vi "ZedBoardWordCalculator.vi"() -> ()   [LabVIEW 2012]
panel:
  in  "Power Pulse\nReject Config":u16
  in  "Power Mon \nAcc Mode":string(combo)
  in  "Power Mon Test Mode":string(combo)
  in  "0       1   ...    Power Mon Chan Enable    ...      9       10     11":bool[](array[boolean])
  out "word9":string
  in  "SoftDEMUX \nSelector Enable":bool
  in  "Sync Select 3B":string(combo)
  in  "Sync Select 2B":string(combo)
  in  "Sync Select 1B":string(combo)
  in  "Sync Select 0B":string(combo)
  in  "Sync Select 7":string(combo)
  in  "Sync Select 6":string(combo)
  in  "Sync Select 5":string(combo)
  in  "Sync Select 4":string(combo)
  in  "Sync Select 3A":string(combo)
  in  "Sync Select 2A":string(combo)
  in  "Sync Select 1A":string(combo)
  in  "Sync Select 0A":string(combo)
  in  "Sync Test\nMode Config":u32
  in  "Pulse Period\n(clock cycles -1)":u32
  in  "Channel DEMUX \nSelector":bool
  in  "Channel \nHold Order":bool
  in  "Channel \nTransfer Order":bool
  in  "Throttle Mode":string(combo)
  in  "Sync Test Mode Select":string(combo)
  in  "Data Input Test Mode":string(combo)
  in  "PIN5 Pulse Durration Ave 2^N":u16
  in  "PIN4 Pulse Durration Ave 2^N":u16
  in  "PIN3 Pulse Durration Ave 2^N":u16
  in  "PIN2 Pulse Durration Ave 2^N":u16
  in  "PIN1 Pulse Durration Ave 2^N":u16
  out "wordA":string
  in  "PIN0 Pulse Durration Ave 2^N":u16
  in  "Sync Input Polarity":bool[](array[boolean])
  in  "DIN Demux Polarity":bool[](array[boolean])
  in  "DIN Polarity":bool[](array[boolean])
  out "word8":string
  out "word7":string
  out "word6":string
  out "word5":string
  out "word4":string
  out "word3":string
  out "word2":string
  out "word1":string
  out "word0":string
  in  "Demux Channel Enable":bool[](array[boolean])
  in  "Relative Time Step":u32
  in  "Time Reset":bool
  in  "Profiles Per Histogram":u16
  in  "Number of Bins":u16
  in  "User Reset":bool
  in  "Counts Per Bin":u16
  in  "0      1       2   ...    Reset Profile Accumulator     ...   10     11":bool[](array[boolean])
  in  "0       1      2    ...     Channel Enable        ...         9      10     11":bool[](array[boolean])
  in  "Sync Enable":bool[](array[boolean])
  in  "stop":bool
  # "word0"
  # "word1"
  # "word2"
  # "word3"
  # "word4"
  # "valid range (2-4096)"
  # "valid range (2-4096)"
  # "valid range (1-32,768)"
  # "word5"
  # "word6"
  # "valid range (0-64)"
  # "valid range (0-256)"
  # "word7"
  # "word8"
  # "word9"
  # "valid range (0-256)"
  # "wordA"
  # "N=valid range (0-15)"
  # "N=valid range (0-15)"
  # "N=valid range (0-15)"
  # "N=valid range (0-15)"
  # "N=valid range (0-15)"
  # "N=valid range (0-15)"
  # "word0"
  # "word1"
  # "word2"
  # "word3"
  # "word4"
  # "valid range (2-4096)"
  # "valid range (2-4096)"
  # "valid range (1-32,768)"
  # "word5"
  # "word6"
  # "valid range (0-256)"
  # "valid range (0-64)"
  # "word7"
  # "word8"
  # "valid range (0-33,554,432)"
  # "word9"
  # "N=valid range (0-15)"
  # "N=valid range (0-15)"
  # "N=valid range (0-15)"
  # "N=valid range (0-15)"
  # "N=valid range (0-15)"
  # "N=valid range (0-15)"
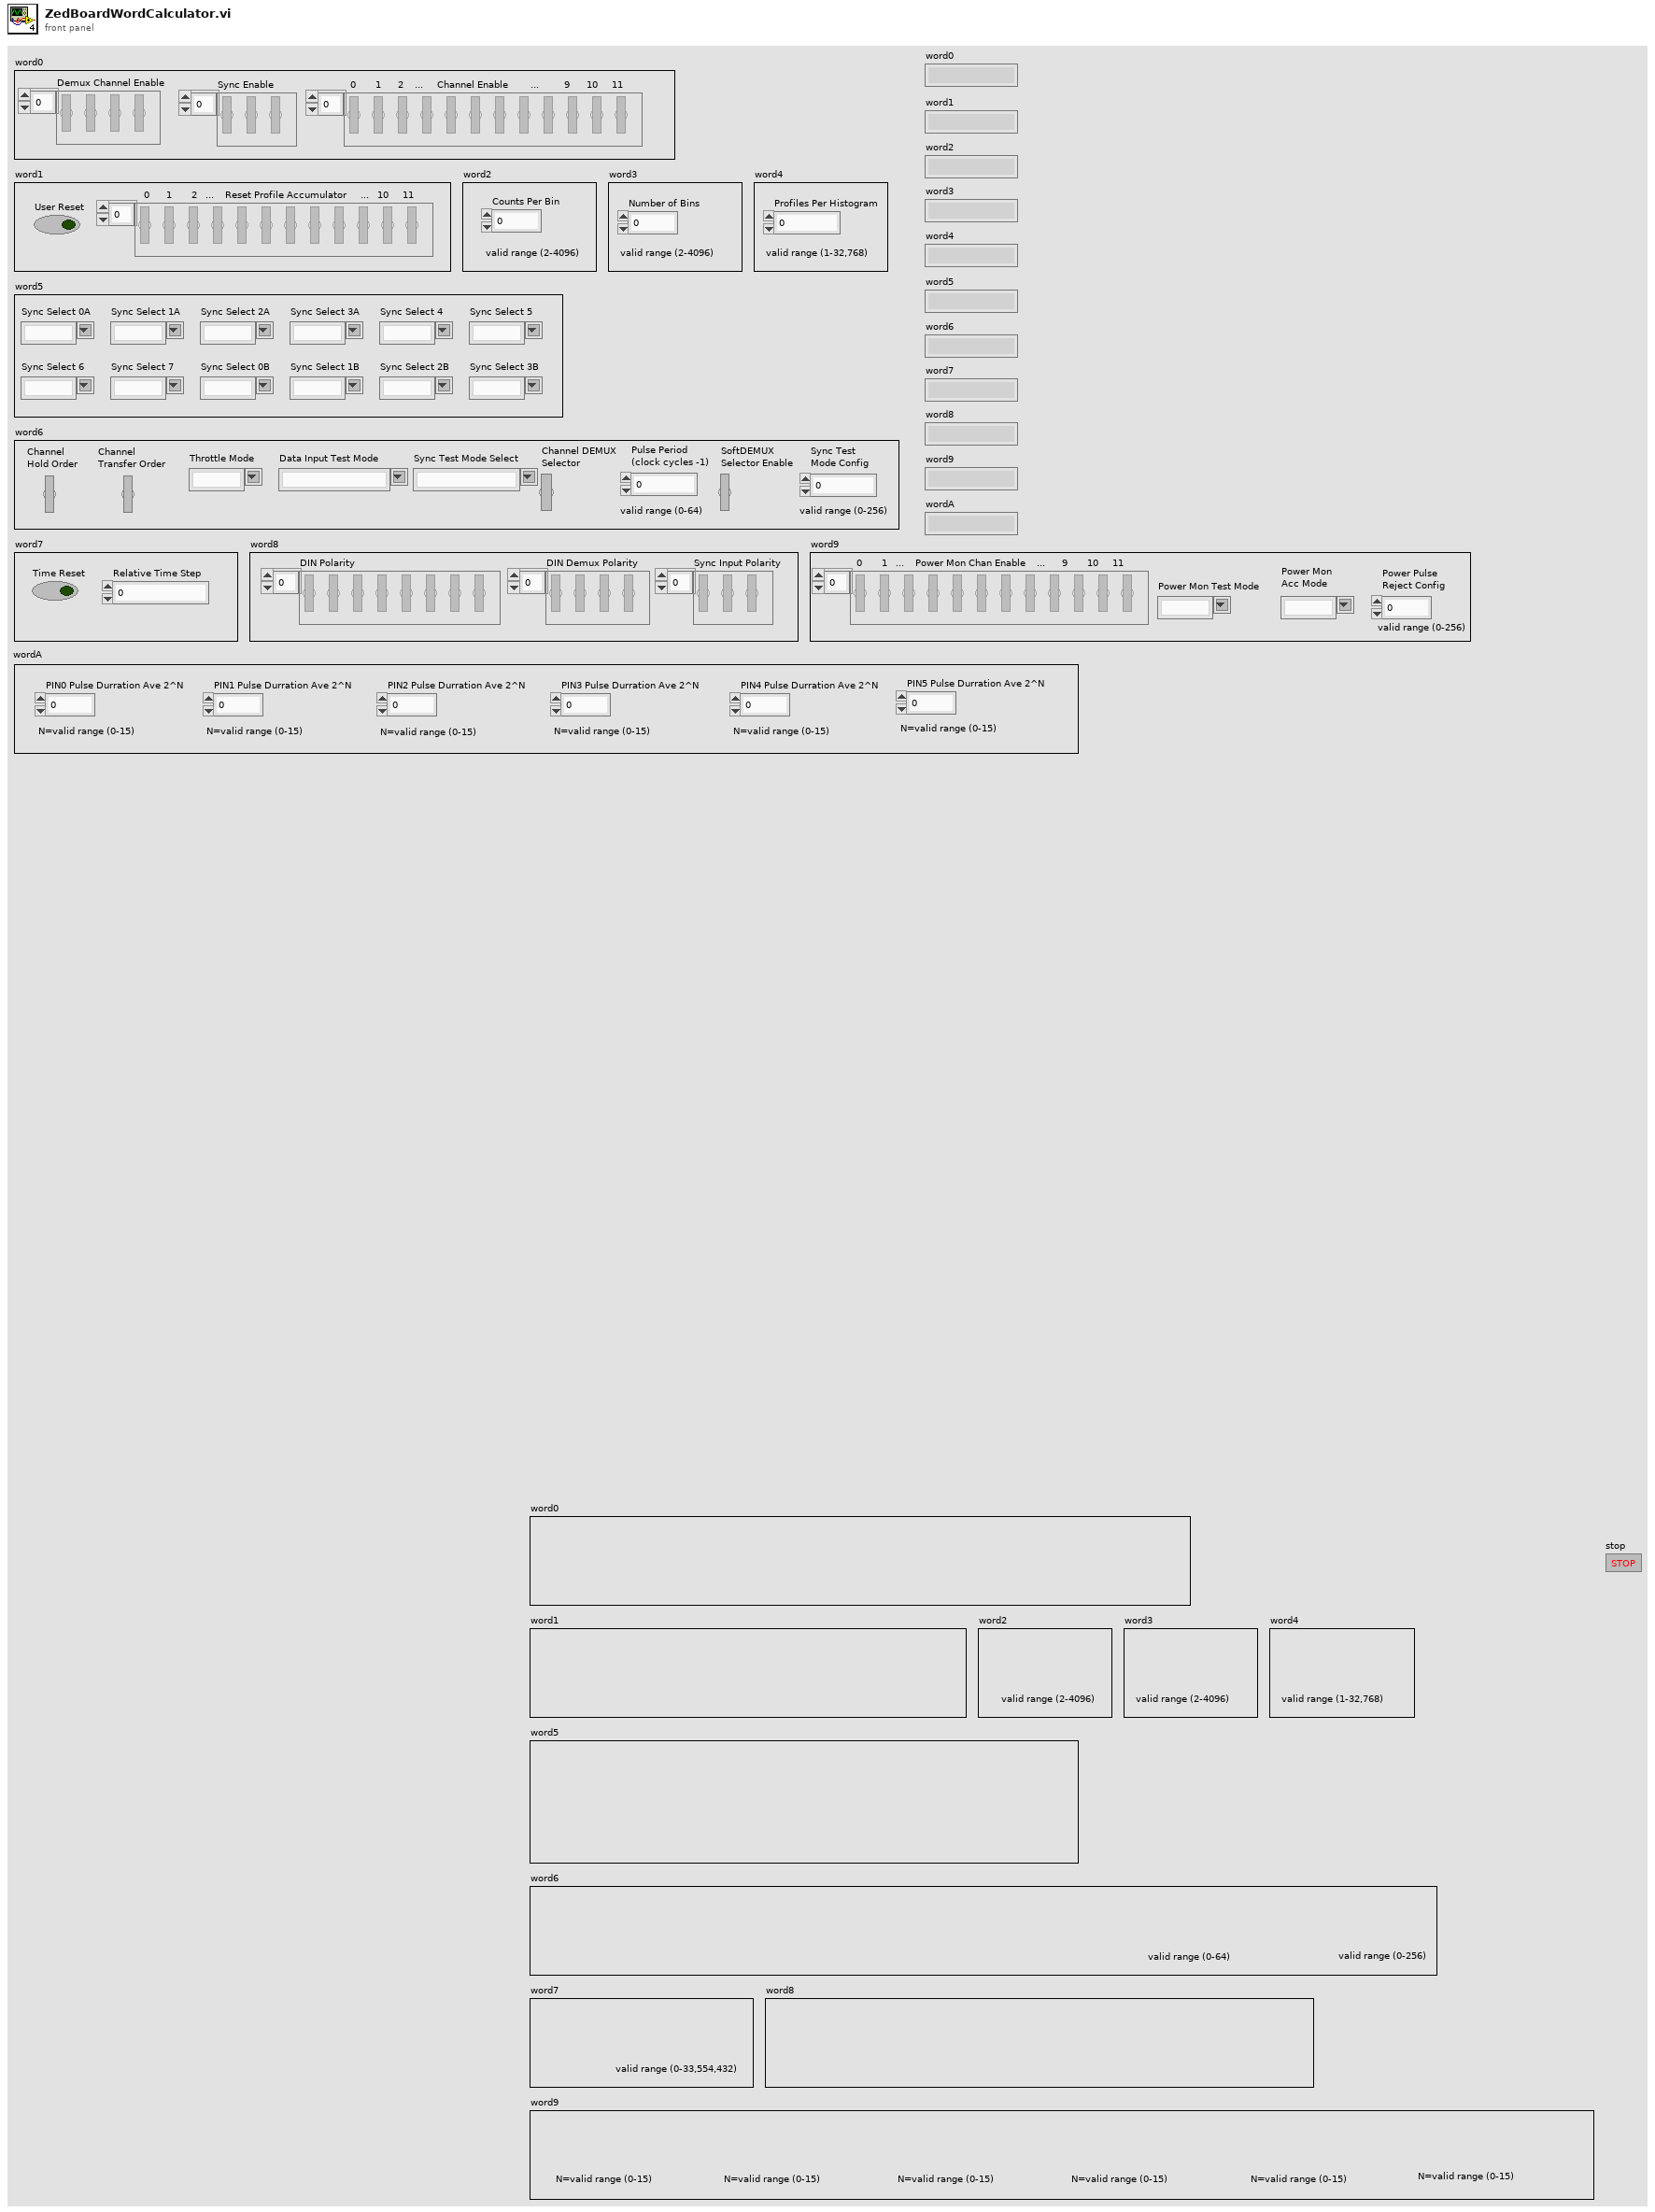
[diagram p1: front panel]
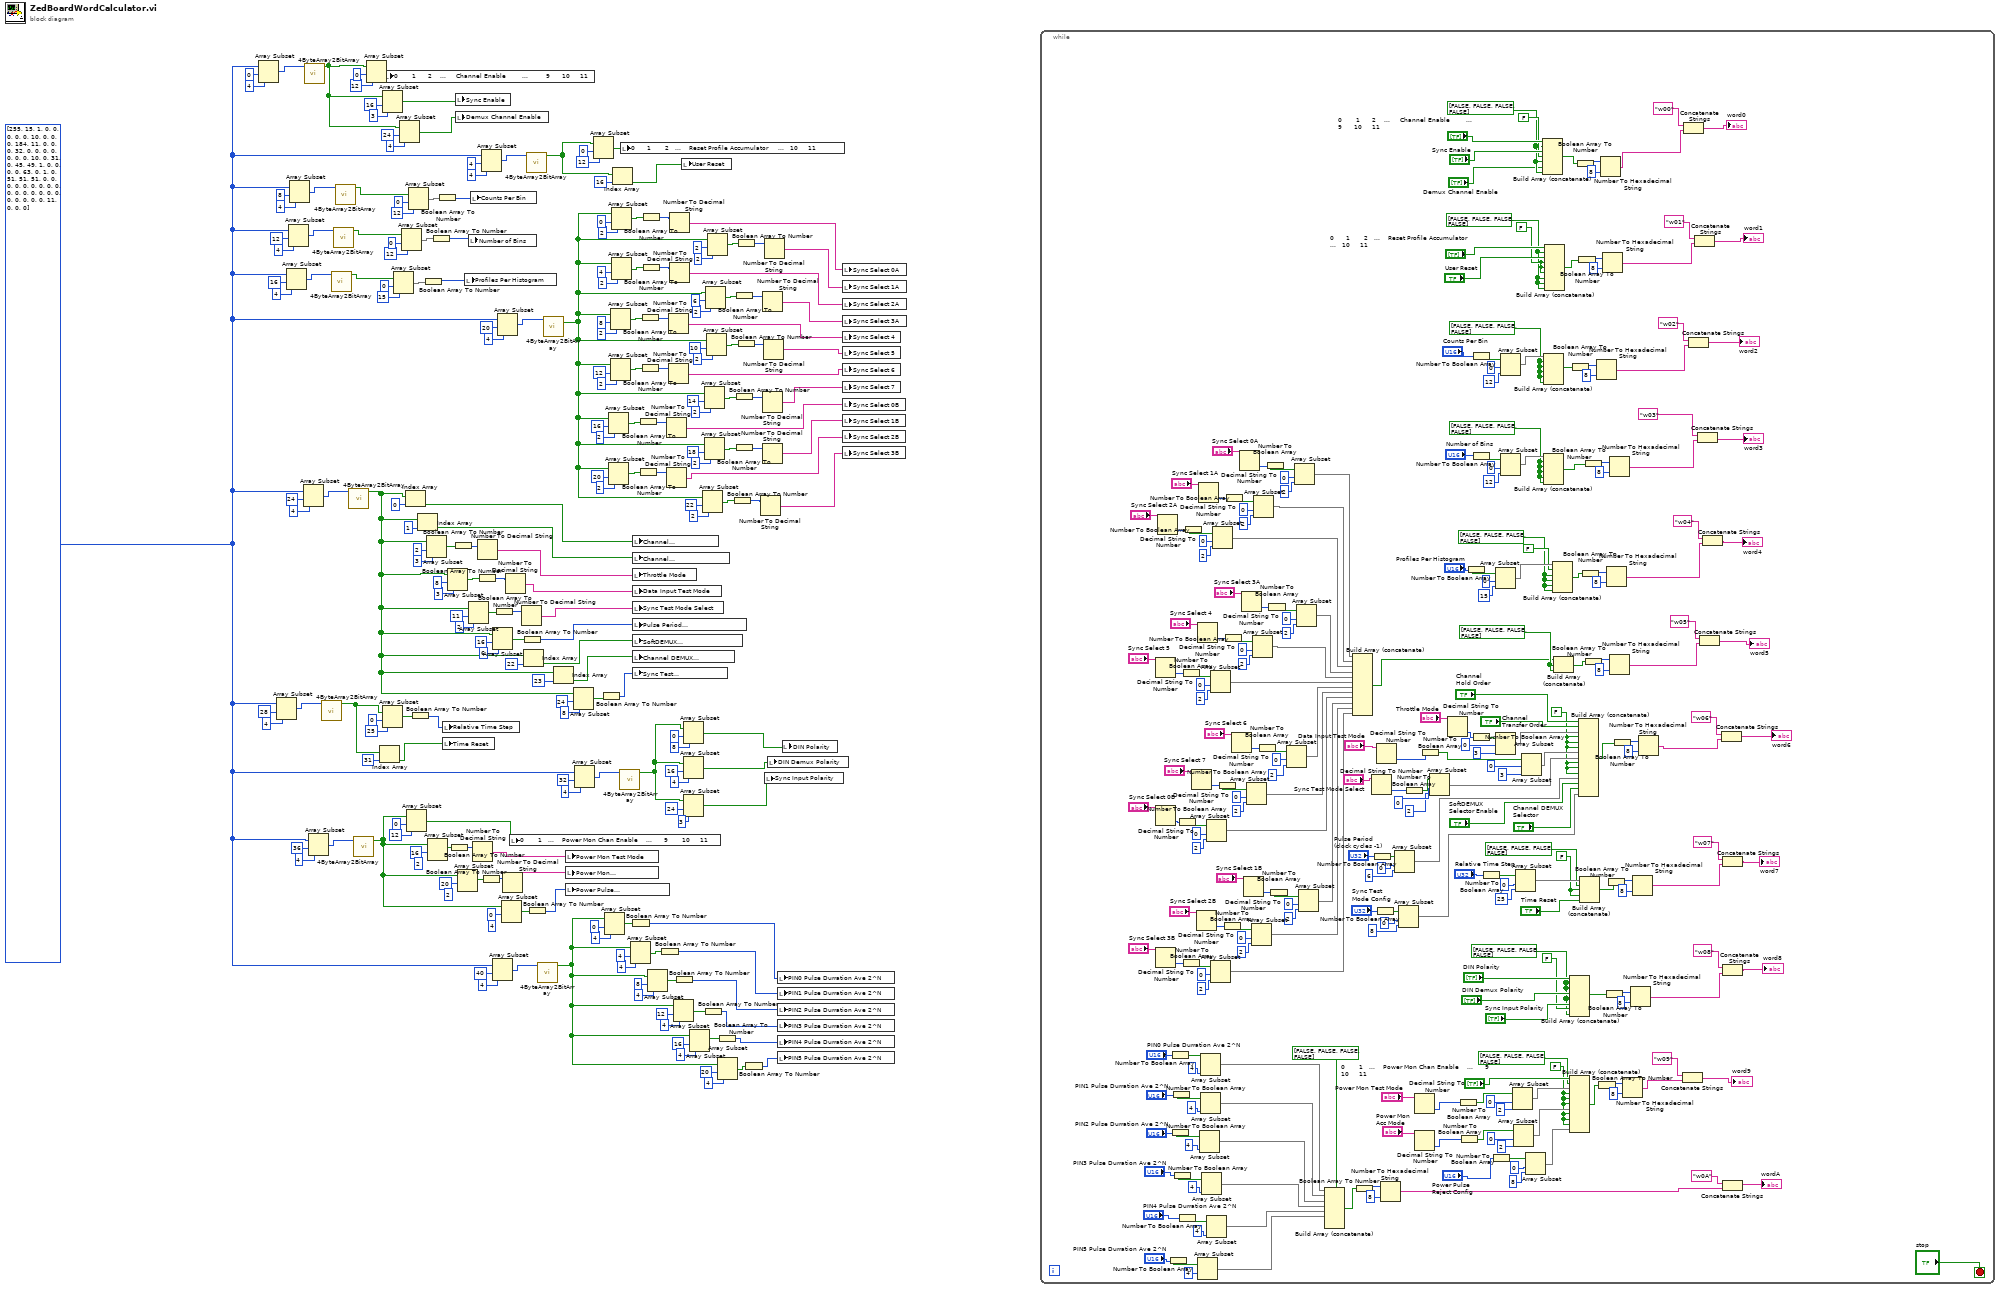
[diagram p0: block diagram]
diagram:
  (unwired) 4 ("length")
  (unwired) 2 ("length")
  (unwired) 2 ("length")
  w1 = u8[] [255, 15, 1, 0, 0, 0, 0, 0, 10, 0, 0, 0, 184, 11, 0, 0, 0, 32, 0, 0, 0, 0, 0, 0, 0, 10, 0, 31, 0, 45, 49, 1, 0, 0, 0, 0, 63, 0, 1, 0, 51, 51, 51, 0, 0, 0, 0, 0, 0, 0, 0, 0, 0, 0, 0, 0, 0, 0, 0, 0, 0, 0, 0, 0, 11, 0, 0, 0] ("subarray")
  n1 = Array Subset(array=w1, index=0, length=4) -> (w183:u8[])
  n2 = Array Subset(array=w1, index=28, length=4) -> (w189:u8[])
  n3 = Array Subset(array=w1, index=16, length=4) -> (w198:u8[])
  n4 = Array Subset(array=w1, index=12, length=4) -> (w201:u8[])
  n5 = Array Subset(array=w1, index=8, length=4) -> (w204:u8[])
  n6 = Array Subset(array=w1, index=24, length=4) -> (w192:u8[])
  n7 = call "4ByteArray2BitArray.vi"("array"=w183) -> ("Array"=w25:bool[])  [unwired: 10 in]
  n8 = Array Subset(array=w1, index=36, length=4) -> (w17:u8[])
  n9 = call "4ByteArray2BitArray.vi"("array"=w189) -> ("Array"=w145:bool[])  [unwired: 10 in]
  n10 = call "4ByteArray2BitArray.vi"("array"=w198) -> ("Array"=w47:bool[])  [unwired: 10 in]
  n11 = call "4ByteArray2BitArray.vi"("array"=w201) -> ("Array"=w42:bool[])  [unwired: 10 in]
  n12 = call "4ByteArray2BitArray.vi"("array"=w204) -> ("Array"=w37:bool[])  [unwired: 10 in]
  n13 = call "4ByteArray2BitArray.vi"("array"=w192) -> ("Array"=w22:bool[])  [unwired: 10 in]
  n14 = call "4ByteArray2BitArray.vi"("array"=w17) -> ("Array"=w3:bool[])  [unwired: 10 in]
  n15 = Array Subset(array=w25, index=0, length=12) -> (w213:bool[])
  n16 = Index Array(array=w145, index=31) -> (element=w143:bool)
  n17 = Array Subset(array=w25, index=16, length=3) -> (w24:bool[])
  n18 = Array Subset(array=w145, index=0, length=25) -> (w141:bool[])
  n19 = local write "0       1      2    ...     Channel Enable        ...         9      10     11"(w213) -> ()
  n20 = Array Subset(array=w47, index=0, length=15) -> (w48:bool[])
  n21 = Array Subset(array=w25, index=24, length=4) -> (w23:bool[])
  n22 = Array Subset(array=w42, index=0, length=12) -> (w43:bool[])
  n23 = Index Array(array=w22, index=0) -> (element=w123:bool)
  n24 = Array Subset(array=w3, index=0, length=12) -> (w14:bool[])
  n25 = Array Subset(array=w37, index=0, length=12) -> (w38:bool[])
  n26 = Boolean Array To Number(Boolean array=w141) -> (number=w142:u32)
  n27 = Index Array(array=w22, index=1) -> (element=w122:bool)
  n28 = Boolean Array To Number(Boolean array=w48) -> (number=w46:u32)
  n29 = Array Subset(array=w22, index=2, length=3) -> (w129:bool[])
  n30 = Array Subset(array=w3, index=16) -> (w12:bool[])  [unwired: 1 in]
  n31 = Boolean Array To Number(Boolean array=w43) -> (number=w41:u32)
  n32 = Boolean Array To Number(Boolean array=w38) -> (number=w36:u32)
  n33 = local write "Relative Time Step"(w142) -> ()
  n34 = local write "Time Reset"(w143) -> ()
  n35 = Array Subset(array=w22, index=8, length=3) -> (w130:bool[])
  n36 = Boolean Array To Number(Boolean array=w12) -> (number=w11:u32)
  n37 = Boolean Array To Number(Boolean array=w129) -> (number=w121:u32)
  n38 = local write "Sync Enable"(w24) -> ()
  n39 = local write "Demux Channel Enable"(w23) -> ()
  n40 = Array Subset(array=w3, index=20) -> (w8:bool[])  [unwired: 1 in]
  n41 = local write "Profiles Per Histogram"(w46) -> ()
  n42 = local write "Number of Bins"(w41) -> ()
  n43 = Array Subset(array=w22, index=11, length=2) -> (w128:bool[])
  n44 = local write "Counts Per Bin"(w36) -> ()
  n45 = Number To Decimal String(number=w11) -> (decimal integer string=w10:string)  [unwired: 1 in]
  n46 = Boolean Array To Number(Boolean array=w130) -> (number=w119:u32)
  n47 = Number To Decimal String(number=w121) -> (decimal integer string=w120:string)  [unwired: 1 in]
  n48 = Array Subset(array=w1, index=4, length=4) -> (w207:u8[])
  n49 = Boolean Array To Number(Boolean array=w8) -> (number=w7:u32)
  n50 = Array Subset(array=w1, index=40, length=4) -> (w210:u8[])
  n51 = Array Subset(array=w22, index=16, length=6) -> (w127:bool[])
  n52 = Boolean Array To Number(Boolean array=w128) -> (number=w117:u32)
  n53 = Array Subset(array=w1, index=20, length=4) -> (w195:u8[])
  n54 = Array Subset(array=w3, index=0) -> (w4:bool[])  [unwired: 1 in]
  n55 = Number To Decimal String(number=w7) -> (decimal integer string=w6:string)  [unwired: 1 in]
  n56 = Number To Decimal String(number=w119) -> (decimal integer string=w118:string)  [unwired: 1 in]
  n57 = local write "0       1   ...    Power Mon Chan Enable    ...      9       10     11"(w14) -> ()
  n58 = Number To Decimal String(number=w117) -> (decimal integer string=w116:string)  [unwired: 1 in]
  n59 = Boolean Array To Number(Boolean array=w127) -> (number=w113:u32)
  n60 = Index Array(array=w22, index=22) -> (element=w20:bool)
  n61 = call "4ByteArray2BitArray.vi"("array"=w207) -> ("Array"=w32:bool[])  [unwired: 10 in]
  n62 = Boolean Array To Number(Boolean array=w4) -> (number=w2:u32)
  n63 = call "4ByteArray2BitArray.vi"("array"=w210) -> ("Array"=w170:bool[])  [unwired: 10 in]
  n64 = call "4ByteArray2BitArray.vi"("array"=w195) -> ("Array"=w63:bool[])  [unwired: 10 in]
  n65 = Index Array(array=w22, index=23) -> (element=w114:bool)
  n66 = local write "Power Mon \nAcc Mode"(w6) -> ()
  n67 = local write "Power Mon Test Mode"(w10) -> ()
  n68 = local write "Power Pulse\nReject Config"(w2) -> ()
  n69 = Array Subset(array=w22, index=24, length=8) -> (w126:bool[])
  n70 = Array Subset(array=w1, index=32, length=4) -> (w186:u8[])
  n71 = Array Subset(array=w32, index=0, length=12) -> (w31:bool[])
  n72 = Boolean Array To Number(Boolean array=w126) -> (number=w112:u32)
  n73 = Array Subset(array=w170, index=0, length=4) -> (w167:bool[])
  n74 = Array Subset(array=w63, index=16, length=2) -> (w77:bool[])
  n75 = Array Subset(array=w63, index=20, length=2) -> (w69:bool[])
  n76 = Array Subset(array=w63, index=8, length=2) -> (w93:bool[])
  n77 = Array Subset(array=w63, index=12, length=2) -> (w85:bool[])
  n78 = Array Subset(array=w63, index=0, length=2) -> (w109:bool[])
  n79 = Array Subset(array=w63, index=4, length=2) -> (w101:bool[])
  n80 = Index Array(array=w32, index=16) -> (element=w30:bool)
  n81 = call "4ByteArray2BitArray.vi"("array"=w186) -> ("Array"=w151:bool[])  [unwired: 10 in]
  n82 = local write "0      1       2   ...    Reset Profile Accumulator     ...   10     11"(w31) -> ()
  n83 = Array Subset(array=w170, index=4, length=4) -> (w169:bool[])
  n84 = Boolean Array To Number(Boolean array=w167) -> (number=w166:u32)
  n85 = local write "Channel \nHold Order"(w123) -> ()
  n86 = local write "Channel \nTransfer Order"(w122) -> ()
  n87 = local write "Throttle Mode"(w120) -> ()
  n88 = local write "Data Input Test Mode"(w118) -> ()
  n89 = local write "Sync Test Mode Select"(w116) -> ()
  n90 = local write "Pulse Period\n(clock cycles -1)"(w113) -> ()
  n91 = local write "SoftDEMUX \nSelector Enable"(w20) -> ()
  n92 = local write "Channel DEMUX \nSelector"(w114) -> ()
  n93 = local write "Sync Test\nMode Config"(w112) -> ()
  n94 = Boolean Array To Number(Boolean array=w77) -> (number=w76:u32)
  n95 = Boolean Array To Number(Boolean array=w69) -> (number=w68:u32)
  n96 = Boolean Array To Number(Boolean array=w93) -> (number=w92:u32)
  n97 = Boolean Array To Number(Boolean array=w85) -> (number=w84:u32)
  n98 = Boolean Array To Number(Boolean array=w109) -> (number=w108:u32)
  n99 = Boolean Array To Number(Boolean array=w101) -> (number=w100:u32)
  n100 = Array Subset(array=w170, index=8, length=4) -> (w164:bool[])
  n101 = Boolean Array To Number(Boolean array=w169) -> (number=w168:u32)
  n102 = Number To Decimal String(number=w76) -> (decimal integer string=w54:string)  [unwired: 1 in]
  n103 = Number To Decimal String(number=w68) -> (decimal integer string=w52:string)  [unwired: 1 in]
  n104 = Number To Decimal String(number=w92) -> (decimal integer string=w58:string)  [unwired: 1 in]
  n105 = Number To Decimal String(number=w84) -> (decimal integer string=w56:string)  [unwired: 1 in]
  n106 = Number To Decimal String(number=w108) -> (decimal integer string=w62:string)  [unwired: 1 in]
  n107 = Number To Decimal String(number=w100) -> (decimal integer string=w60:string)  [unwired: 1 in]
  n108 = Array Subset(array=w170, index=12, length=4) -> (w163:bool[])
  n109 = Boolean Array To Number(Boolean array=w164) -> (number=w165:u32)
  n110 = local write "User Reset"(w30) -> ()
  n111 = Array Subset(array=w151, index=16, length=4) -> (w148:bool[])
  n112 = Array Subset(array=w151, index=24, length=3) -> (w149:bool[])
  n113 = Array Subset(array=w151, index=0, length=8) -> (w150:bool[])
  n114 = Array Subset(array=w170, index=16, length=4) -> (w162:bool[])
  n115 = Array Subset(array=w63, index=22, length=2) -> (w65:bool[])
  n116 = Boolean Array To Number(Boolean array=w163) -> (number=w158:u32)
  n117 = Array Subset(array=w63, index=14, length=2) -> (w81:bool[])
  n118 = Array Subset(array=w63, index=18, length=2) -> (w73:bool[])
  n119 = Array Subset(array=w63, index=6, length=2) -> (w97:bool[])
  n120 = Array Subset(array=w63, index=10, length=2) -> (w89:bool[])
  n121 = Array Subset(array=w63, index=2, length=2) -> (w105:bool[])
  n122 = Boolean Array To Number(Boolean array=w162) -> (number=w159:u32)
  n123 = Array Subset(array=w170, index=20, length=4) -> (w161:bool[])
  n124 = Boolean Array To Number(Boolean array=w65) -> (number=w64:u32)
  n125 = Boolean Array To Number(Boolean array=w81) -> (number=w80:u32)
  n126 = Boolean Array To Number(Boolean array=w73) -> (number=w72:u32)
  n127 = Boolean Array To Number(Boolean array=w97) -> (number=w96:u32)
  n128 = Boolean Array To Number(Boolean array=w89) -> (number=w88:u32)
  n129 = Boolean Array To Number(Boolean array=w105) -> (number=w104:u32)
  n130 = Boolean Array To Number(Boolean array=w161) -> (number=w160:u32)
  n131 = Number To Decimal String(number=w64) -> (decimal integer string=w51:string)  [unwired: 1 in]
  n132 = Number To Decimal String(number=w80) -> (decimal integer string=w55:string)  [unwired: 1 in]
  n133 = Number To Decimal String(number=w72) -> (decimal integer string=w53:string)  [unwired: 1 in]
  n134 = Number To Decimal String(number=w96) -> (decimal integer string=w59:string)  [unwired: 1 in]
  n135 = Number To Decimal String(number=w88) -> (decimal integer string=w57:string)  [unwired: 1 in]
  n136 = Number To Decimal String(number=w104) -> (decimal integer string=w61:string)  [unwired: 1 in]
  n137 = local write "Sync Input Polarity"(w149) -> ()
  n138 = local write "DIN Demux Polarity"(w148) -> ()
  n139 = local write "PIN0 Pulse Durration Ave 2^N"(w166) -> ()
  n140 = local write "PIN1 Pulse Durration Ave 2^N"(w168) -> ()
  n141 = local write "PIN2 Pulse Durration Ave 2^N"(w165) -> ()
  n142 = local write "PIN3 Pulse Durration Ave 2^N"(w158) -> ()
  n143 = local write "PIN4 Pulse Durration Ave 2^N"(w159) -> ()
  n144 = local write "PIN5 Pulse Durration Ave 2^N"(w160) -> ()
  n145 = local write "DIN Polarity"(w150) -> ()
  n146 = local write "Sync Select 0A"(w62) -> ()
  n147 = local write "Sync Select 1A"(w61) -> ()
  n148 = local write "Sync Select 2A"(w60) -> ()
  n149 = local write "Sync Select 3A"(w59) -> ()
  n150 = local write "Sync Select 4"(w58) -> ()
  n151 = local write "Sync Select 5"(w57) -> ()
  n152 = local write "Sync Select 6"(w56) -> ()
  n153 = local write "Sync Select 7"(w55) -> ()
  n154 = local write "Sync Select 0B"(w54) -> ()
  n155 = local write "Sync Select 1B"(w53) -> ()
  n156 = local write "Sync Select 2B"(w52) -> ()
  n157 = local write "Sync Select 3B"(w51) -> ()
  n158 = while {
    stop <- "stop" stop-if-true
    w232 = FALSE ("Read Register")
    w408 = bool[] [FALSE, FALSE, FALSE, FALSE] ("appended array")
    w432 = bool[] [FALSE, FALSE, FALSE, FALSE] ("appended array")
    w438 = FALSE ("Read Register")
    w375 = FALSE ("Read Register")
    w443 = bool[] [FALSE, FALSE, FALSE, FALSE] ("appended array")
    w296 = bool[] [FALSE, FALSE, FALSE, FALSE] ("appended array")
    w441 = bool[] [FALSE, FALSE, FALSE, FALSE] ("appended array")
    w442 = bool[] [FALSE, FALSE, FALSE, FALSE] ("appended array")
    w456 = FALSE ("Read Register")
    w455 = bool[] [FALSE, FALSE, FALSE, FALSE] ("appended array")
    w460 = bool[] [FALSE, FALSE, FALSE, FALSE] ("appended array")
    n159 = Decimal String To Number(string="Sync Select 5") -> (number=w340:i32)  [unwired: 2 in, 1 out]
    n160 = Decimal String To Number(string="Sync Select 0B") -> (number=w325:i32)  [unwired: 2 in, 1 out]
    n161 = Decimal String To Number(string="Sync Select 3B") -> (number=w310:i32)  [unwired: 2 in, 1 out]
    n162 = Decimal String To Number(string="Sync Select 2A") -> (number=w355:i32)  [unwired: 2 in, 1 out]
    n163 = Number To Boolean Array(number="PIN5 Pulse Durration Ave 2^N") -> (Boolean array=w424:bool[])
    n164 = Number To Boolean Array(number="PIN0 Pulse Durration Ave 2^N") -> (Boolean array=w430:bool[])
    n165 = Number To Boolean Array(number="PIN2 Pulse Durration Ave 2^N") -> (Boolean array=w420:bool[])
    n166 = Number To Boolean Array(number="PIN1 Pulse Durration Ave 2^N") -> (Boolean array=w428:bool[])
    n167 = Number To Boolean Array(number="PIN3 Pulse Durration Ave 2^N") -> (Boolean array=w422:bool[])
    n168 = Number To Boolean Array(number=w325) -> (Boolean array=w327:bool[])
    n169 = Number To Boolean Array(number="PIN4 Pulse Durration Ave 2^N") -> (Boolean array=w426:bool[])
    n170 = Number To Boolean Array(number=w340) -> (Boolean array=w342:bool[])
    n171 = Number To Boolean Array(number=w310) -> (Boolean array=w312:bool[])
    n172 = Number To Boolean Array(number=w355) -> (Boolean array=w357:bool[])
    n173 = Decimal String To Number(string="Sync Select 7") -> (number=w330:i32)  [unwired: 2 in, 1 out]
    n174 = Decimal String To Number(string="Sync Select 2B") -> (number=w315:i32)  [unwired: 2 in, 1 out]
    n175 = Decimal String To Number(string="Sync Select 4") -> (number=w345:i32)  [unwired: 2 in, 1 out]
    n176 = Array Subset(array=w424, length=4) -> (w409:bool[])  [unwired: 1 in]
    n177 = Decimal String To Number(string="Sync Select 1A") -> (number=w360:i32)  [unwired: 2 in, 1 out]
    n178 = Array Subset(array=w420, length=4) -> (w412:bool[])  [unwired: 1 in]
    n179 = Array Subset(array=w430, length=4) -> (w414:bool[])  [unwired: 1 in]
    n180 = Array Subset(array=w428, length=4) -> (w413:bool[])  [unwired: 1 in]
    n181 = Array Subset(array=w422, length=4) -> (w411:bool[])  [unwired: 1 in]
    n182 = Array Subset(array=w327, index=0, length=2) -> (w300:bool[])
    n183 = Array Subset(array=w426, length=4) -> (w410:bool[])  [unwired: 1 in]
    n184 = Array Subset(array=w342, index=0, length=2) -> (w304:bool[])
    n185 = Array Subset(array=w312, index=0, length=2) -> (w303:bool[])
    n186 = Array Subset(array=w357, index=0, length=2) -> (w307:bool[])
    n187 = Number To Boolean Array(number=w330) -> (Boolean array=w332:bool[])
    n188 = Number To Boolean Array(number=w315) -> (Boolean array=w317:bool[])
    n189 = Number To Boolean Array(number=w345) -> (Boolean array=w347:bool[])
    n190 = Number To Boolean Array(number=w360) -> (Boolean array=w362:bool[])
    n191 = Decimal String To Number(string="Sync Select 6") -> (number=w335:i32)  [unwired: 2 in, 1 out]
    n192 = Decimal String To Number(string="Sync Select 0A") -> (number=w365:i32)  [unwired: 2 in, 1 out]
    n193 = Decimal String To Number(string="Sync Select 3A") -> (number=w350:i32)  [unwired: 2 in, 1 out]
    n194 = Decimal String To Number(string="Sync Select 1B") -> (number=w320:i32)  [unwired: 2 in, 1 out]
    n195 = Array Subset(array=w332, index=0, length=2) -> (w299:bool[])
    n196 = Array Subset(array=w317, index=0, length=2) -> (w302:bool[])
    n197 = Array Subset(array=w347, index=0, length=2) -> (w305:bool[])
    n198 = Array Subset(array=w362, index=0, length=2) -> (w308:bool[])
    n199 = Number To Boolean Array(number=w335) -> (Boolean array=w337:bool[])
    n200 = Number To Boolean Array(number=w365) -> (Boolean array=w367:bool[])
    n201 = Number To Boolean Array(number=w350) -> (Boolean array=w352:bool[])
    n202 = Number To Boolean Array(number=w320) -> (Boolean array=w322:bool[])
    n203 = Array Subset(array=w337, index=0, length=2) -> (w298:bool[])
    n204 = Array Subset(array=w367, index=0, length=2) -> (w309:bool[])
    n205 = Array Subset(array=w352, index=0, length=2) -> (w306:bool[])
    n206 = Array Subset(array=w322, index=0, length=2) -> (w301:bool[])
    n207 = Build Array (concatenate)(w414, w413, w412, w411, w410, w409, w408, w408) -> (w257:bool[])
    n208 = Build Array (concatenate)(w309, w308, w307, w306, w305, w304, w298, w299, w300, w301, w302, w303) -> (w397:bool[])
    n209 = Boolean Array To Number(Boolean array=w257) -> (number=w275:u32)
    n210 = Decimal String To Number(string="Sync Test Mode Select") -> (number=w391:i32)  [unwired: 2 in, 1 out]
    n211 = Number To Boolean Array(number="Pulse Period\n(clock cycles -1)") -> (Boolean array=w384:bool[])
    n212 = Number To Boolean Array(number="Sync Test\nMode Config") -> (Boolean array=w374:bool[])
    n213 = Decimal String To Number(string="Data Input Test Mode") -> (number=w392:i32)  [unwired: 2 in, 1 out]
    n214 = Number To Hexadecimal String(1:i16 8 ("width (-)"), 2:w275) -> (0:w256:string)
    n215 = Array Subset(array=w384, index=0, length=6) -> (w254:bool[])
    n216 = Array Subset(array=w374, index=0, length=8) -> (w255:bool[])
    n217 = Number To Boolean Array(number=w391) -> (Boolean array=w385:bool[])
    n218 = Decimal String To Number(string="Power Mon Test Mode") -> (number=w243:i32)  [unwired: 2 in, 1 out]
    n219 = Decimal String To Number(string="Power Mon \nAcc Mode") -> (number=w238:i32)  [unwired: 2 in, 1 out]
    n220 = Number To Boolean Array(number=w392) -> (Boolean array=w386:bool[])
    n221 = Array Subset(array=w385, index=0, length=2) -> (w376:bool[])
    n222 = Decimal String To Number(string="Throttle Mode") -> (number=w395:i32)  [unwired: 2 in, 1 out]
    n223 = Number To Boolean Array(number=w243) -> (Boolean array=w242:bool[])
    n224 = Number To Boolean Array(number=w238) -> (Boolean array=w237:bool[])
    n225 = Number To Boolean Array(number="Profiles Per Histogram") -> (Boolean array=w446:bool[])
    n226 = Number To Boolean Array(number=w395) -> (Boolean array=w469:bool[])
    n227 = Number To Boolean Array(number="Counts Per Bin") -> (Boolean array=w472:bool[])
    n228 = Number To Boolean Array(number="Number of Bins") -> (Boolean array=w451:bool[])
    n229 = Number To Boolean Array(number="Relative Time Step") -> (Boolean array=w466:bool[])
    n230 = Number To Boolean Array(number="Power Pulse\nReject Config") -> (Boolean array=w230:bool[])
    n231 = Array Subset(array=w446, index=0, length=15) -> (w445:bool[])
    n232 = Array Subset(array=w469, index=0, length=3) -> (w380:bool[])
    n233 = Array Subset(array=w472, index=0, length=12) -> (w454:bool[])
    n234 = Array Subset(array=w451, index=0, length=12) -> (w450:bool[])
    n235 = Array Subset(array=w242, index=0, length=2) -> (w239:bool[])
    n236 = Array Subset(array=w237, index=0, length=2) -> (w233:bool[])
    n237 = Array Subset(array=w466, index=0, length=25) -> (w440:bool[])
    n238 = Array Subset(array=w386, index=0, length=3) -> (w377:bool[])
    n239 = Array Subset(array=w230, index=0, length=8) -> (w227:bool[])
    n240 = Build Array (concatenate)("0       1      2    ...     Channel Enable        ...         9      10     11", w460, "Sync Enable", FALSE ("Read Register"), w460, "Demux Channel Enable", w460) -> (w273:bool[])
    n241 = Build Array (concatenate)(w454, w442, w442, w442, w442, w442) -> (w269:bool[])
    n242 = Build Array (concatenate)(w450, w441, w441, w441, w441, w441) -> (w292:bool[])
    n243 = Build Array (concatenate)("0      1       2   ...    Reset Profile Accumulator     ...   10     11", w455, "User Reset", w456, w456, w456, w455, w455, w455) -> (w271:bool[])
    n244 = Build Array (concatenate)(w445, FALSE ("Read Register"), w296, w296, w296, w296) -> (w267:bool[])
    n245 = Build Array (concatenate)(w397, w443, w443) -> (w265:bool[])
    n246 = Build Array (concatenate)("0       1   ...    Power Mon Chan Enable    ...      9       10     11", bool[] [FALSE, FALSE, FALSE, FALSE] ("appended array"), w239, w232, w232, w232, w233, w232, w232, w232, w227) -> (w247:bool[])
    n247 = Build Array (concatenate)("DIN Polarity", w432, w432, "DIN Demux Polarity", w432, "Sync Input Polarity", FALSE ("Read Register"), w432) -> (w259:bool[])
    n248 = Boolean Array To Number(Boolean array=w269) -> (number=w287:u32)
    n249 = Boolean Array To Number(Boolean array=w273) -> (number=w291:u32)
    n250 = Boolean Array To Number(Boolean array=w271) -> (number=w289:u32)
    n251 = Build Array (concatenate)("Channel \nHold Order", "Channel \nTransfer Order", w380, w375, w375, w375, w377, w376, w375, w375, w375, w254, "SoftDEMUX \nSelector Enable", "Channel DEMUX \nSelector", w255) -> (w263:bool[])
    n252 = Build Array (concatenate)(w440, bool[] [FALSE, FALSE, FALSE, FALSE] ("appended array"), w438, w438, "Time Reset") -> (w261:bool[])
    n253 = Boolean Array To Number(Boolean array=w267) -> (number=w285:u32)
    n254 = Boolean Array To Number(Boolean array=w292) -> (number=w295:u32)
    n255 = Boolean Array To Number(Boolean array=w265) -> (number=w283:u32)
    n256 = Number To Hexadecimal String(1:i16 8 ("width (-)"), 2:w287) -> (0:w268:string)
    n257 = Boolean Array To Number(Boolean array=w247) -> (number=w250:u32)
    n258 = Number To Hexadecimal String(1:i16 8 ("width (-)"), 2:w291) -> (0:w272:string)
    n259 = Number To Hexadecimal String(1:i16 8 ("width (-)"), 2:w289) -> (0:w270:string)
    n260 = Boolean Array To Number(Boolean array=w259) -> (number=w277:u32)
    n261 = Number To Hexadecimal String(1:i16 8 ("width (-)"), 2:w285) -> (0:w266:string)
    n262 = Boolean Array To Number(Boolean array=w261) -> (number=w279:u32)
    n263 = Number To Hexadecimal String(1:i16 8 ("width (-)"), 2:w295) -> (0:w293:string)
    n264 = Number To Hexadecimal String(1:i16 8 ("width (-)"), 2:w283) -> (0:w264:string)
    n265 = Boolean Array To Number(Boolean array=w263) -> (number=w281:u32)
    n266 = Number To Hexadecimal String(1:i16 8 ("width (-)"), 2:w250) -> (0:w248:string)
    n267 = Number To Hexadecimal String(1:i16 8 ("width (-)"), 2:w277) -> (0:w258:string)
    n268 = Number To Hexadecimal String(1:i16 8 ("width (-)"), 2:w279) -> (0:w260:string)
    n269 = Number To Hexadecimal String(1:i16 8 ("width (-)"), 2:w281) -> (0:w262:string)
    n270 = Concatenate Strings("w09" ("string"), w248) -> (→"word9":string)
    n271 = Concatenate Strings("w00" ("string"), w272) -> (→"word0":string)
    n272 = Concatenate Strings("w02" ("string"), w268) -> (→"word2":string)
    n273 = Concatenate Strings("w01" ("string"), w270) -> (→"word1":string)
    n274 = Concatenate Strings("w03" ("string"), w293) -> (→"word3":string)
    n275 = Concatenate Strings("w05" ("string"), w264) -> (→"word5":string)
    n276 = Concatenate Strings("w04" ("string"), w266) -> (→"word4":string)
    n277 = Concatenate Strings("w06" ("string"), w262) -> (→"word6":string)
    n278 = Concatenate Strings("w0A" ("string"), w256) -> (→"wordA":string)
    n279 = Concatenate Strings("w07" ("string"), w260) -> (→"word7":string)
    n280 = Concatenate Strings("w08" ("string"), w258) -> (→"word8":string)
  }
